vi "StartTest.vi"() -> ()   [LabVIEW 2016, in "DronaTest.lvlib"]
uses:
  DronaTest.lvlib
  <vilib>/addons/_JKI Toolkits/Caraya/classes/Test/Test.lvclass
panel:
  out "error out":errorcluster
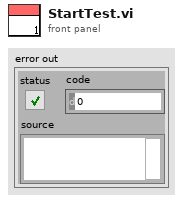
[diagram p1: front panel]
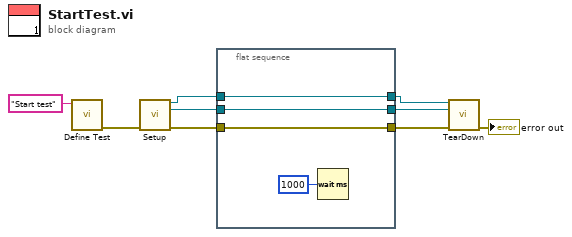
[diagram p0: block diagram]
diagram:
  n1 = call <vilib>:"Define Test.vi"("Label (VI Title)"="Start test") -> ("error out"=w8:errorcluster)  [unwired: 10 in]
  n2 = call "Setup.vi"("error in (no error)"=w8) -> ("Application Ref"=w3:refnum<vi>, "VI out"=w5:refnum<vi>, "error out"=w7:errorcluster)  [unwired: 12 in]
  n3 = flat-sequence {
    tunnel: w7 -> [w12]
    tunnel: [w12] -> w6
    tunnel: [w11] -> w4
    tunnel: w5 -> [w11]
    tunnel: w3 -> [w10]
    tunnel: [w10] -> w2
    frame #0 {
      n4 = Wait (ms)(milliseconds to wait=u32 1000) -> ()  [unwired: 1 out]
    }
  }
  n5 = call "TearDown.vi"("Application Ref"=w2, "VI in"=w4, "error in (no error)"=w6) -> ("error out"=→"error out":errorcluster)  [unwired: 12 in]
